vi "Motor-SetName.vi"(2 "Name":string, 3 "Motor":string="PI1-M2-THETA", 9 "error in (no error)":errorcluster) -> (6 "error out":errorcluster)   [LabVIEW 2009]
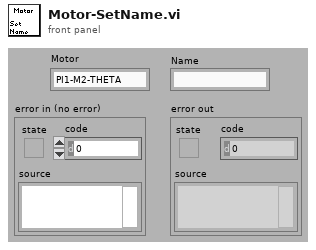
[diagram p1: front panel]
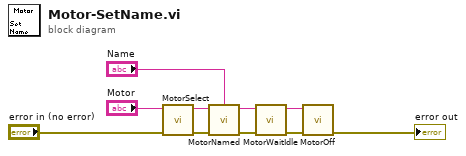
[diagram p0: block diagram]
diagram:
  n1 = call "MotorSelect.vi"("Motor"="Motor", "error in (no error)"="error in (no error)") -> ("Motor out"=w10:string, "error out"=w5:errorcluster)  [unwired: 6 out]
  n2 = call "MotorNamed.vi"("Name"="Name", "Motor in"=w10, "error in (no error)"=w5) -> ("Motor out"=w3:string, "error out"=w4:errorcluster)  [unwired: 1 in, 4 out]
  n3 = call "MotorWaitIdle.vi"("Motor"=w3, "error in (no error)"=w4) -> ("Motor out"=w6:string, "error out"=w7:errorcluster)  [unwired: 6 out]
  n4 = call "MotorOff.vi"("Motor"=w6, "error in (no error)"=w7) -> ("error out"=→"error out":errorcluster)  [unwired: 7 out]
